vi "Close MeasurementLink Session.vi"(8 "error in":errorcluster, 9 "close session behavior":T1, 10 "session in":variant, 11 "instrument in":refnum<class "Instrument.lvclass">) -> (0 "error out":errorcluster)   [LabVIEW 2020, in "MeasurementLink niDigital.lvlib" / "Instrument.lvclass"]
uses:
  Instrument.lvclass
  MeasurementLink Instrument/IInstrument/Close Session Behavior.ctl
  MeasurementLink Measurement Server/Helpers/Error Strings Global Internal.vi
  MeasurementLink Instrument/IInstrument/IInstrument.lvclass
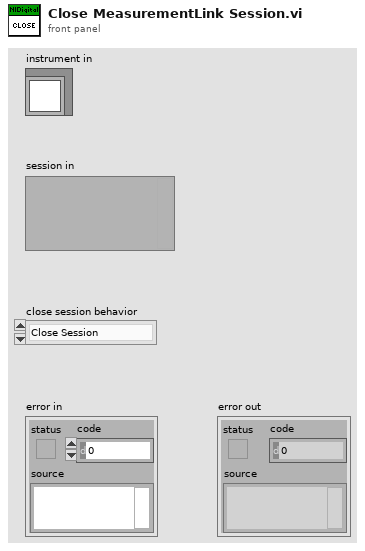
[diagram p1: front panel]
types:
  T1 = typedef "MeasurementLink Instrument.lvlib/IInstrument.lvclass/Close Session Behavior.ctl" = enum16{"Close Session", "Detach Session"}
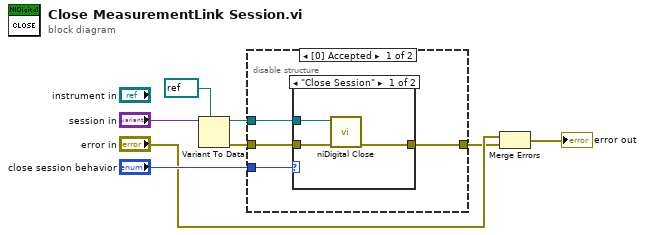
[diagram p0: block diagram]
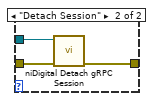
[diagram p2: hidden frame]
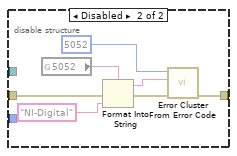
[diagram p3: hidden frame]
diagram:
  n1 = Variant To Data(type=refnum<k15> refnum ("instrument handle"), Variant="session in") -> (data=w5:refnum<k15>, error out=w6:errorcluster)  [unwired: 1 in]
  n2 = disable-structure shown="[0] Accepted" {
    disable-tunnel: "close session behavior" -> [w12 _]
    disable-tunnel: w6 -> [w11 w19]
    disable-tunnel: w5 -> [w10 _]
    disable-tunnel: [w9 w25] -> w1
    frame Enabled {
      n3 = case shown="\"Close Session\"" w12 {
        tunnel: w11 -> [w15 w18]
        tunnel: w10 -> [w14 w16]
        tunnel: [w13 w17] -> w9
        frame "Close Session" {
          n4 = call <instrlib>:"niDigital Close.vi"("instrument handle"=w14, "error in"=w15) -> ("error out"=w13:errorcluster)  [unwired: 13 in]
        }
        frame "Detach Session" {
          n5 = call <instrlib>:"niDigital Detach gRPC Session.vi"("instrument handle"=w16, "error in"=w18) -> ("error out"=w17:errorcluster)  [unwired: 13 in]
        }
      }
    }
    frame Disabled {
      n6 = global read "Error Strings Global Internal.vi" "5052"() -> (w23:string)
      n7 = Format Into String(format string=w23, error in=w19, "NI-Digital") -> (resulting string=w20:string, error out=w21:errorcluster)  [unwired: 1 in]
      n8 = call <vilib>:"Error Cluster From Error Code.vi"("error in (no error)"=w21, "error message (\"\")"=w20, "error code (0)"=5052) -> ("error out"=w25:errorcluster)  [unwired: 6 in]
    }
  }
  n9 = Merge Errors("error in", w1) -> (→"error out":errorcluster)
